vi "Handle Exit.vi"(8 "error in (no error)":errorcluster, 9 "Stop Argument":T1, 10 "Module Admin in":refnum<class "Delacor_lib_QMH_Cloneable Module Admin.lvclass">, 11 "VI reference":refnum<vi>) -> (0 "error out":errorcluster, 3 "Wait for Stop?":bool)   [LabVIEW 2020, in "Counters.lvlib"]
doc: "This VI handles the Exit Message for a DQMH Cloneable module. \n\nThis VI determines if the message was received via the Stop Request or not. If the Exit message was received via the Request Event to Stop the module then there is no need to send the Stop Request again. If it was not, then the Stop Request needs to be fired so the Event Handling Loop can stop.\n\nThis VI also hides the Main.vi Front Panel, this is to ensure that the module stays in memory until the very last step in the Main.vi which is to close the front panel.\n\n_____\nBased on DQMH Project Template 6.1.0.94."
uses:
  Counters.lvlib
  Stop Argument--cluster.ctl
  <vilib>/Delacor/Delacor QMH/Libraries/Cloneable Module Admin_class/Delacor_lib_QMH_Cloneable Module Admin.lvclass
  C:/Program Files (x86)/National Instruments/LabVIEW 2020/vi.lib/Delacor/Delacor QMH/Libraries/Module Admin_class/Delacor_lib_QMH_Module Admin.lvclass
  <vilib>/Delacor/Delacor QMH/Libraries/Cloneable Module Admin_class/Delacor_lib_QMH_Cloneable Module Admin.lvclass/Delacor_lib_QMH_Cloneable Module Admin.ctl
  <vilib>/Delacor/Delacor QMH/Libraries/Module Admin_class/Delacor_lib_QMH_Module Admin.lvclass/Delacor_lib_QMH_Module Admin.ctl
  <vilib>/Delacor/Delacor QMH/Libraries/Cloneable Module Admin_class/Delacor_lib_QMH_Get Module ID.vi
  <vilib>/Delacor/Delacor QMH/Libraries/Module Admin_class/Delacor_lib_QMH_Get External Launch.vi
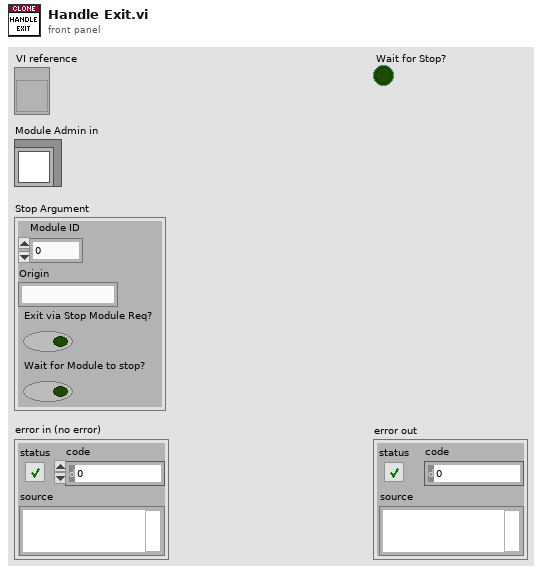
[diagram p1: front panel]
types:
  T1 = typedef "Counters.lvlib/Stop Argument--cluster.ctl" = cluster{"Module ID":i32, "Origin":string, "Exit via Stop Module Req?":bool, "Wait for Module to stop?":bool}
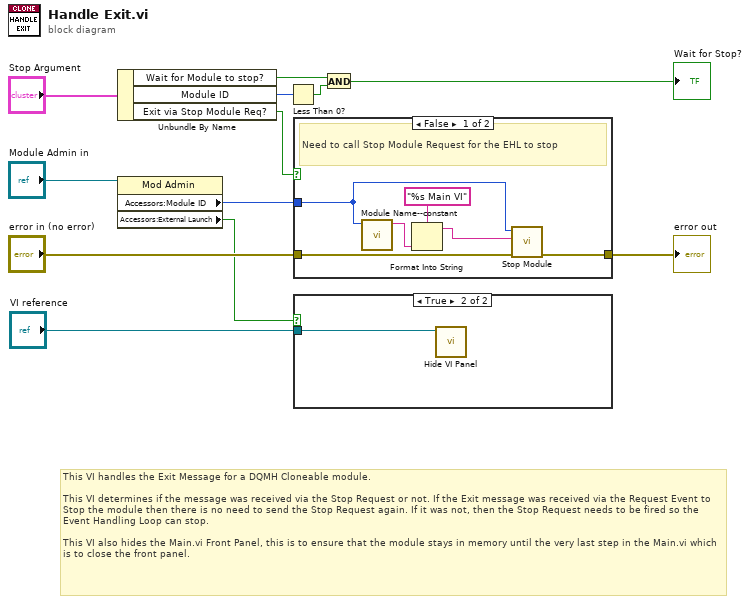
[diagram p0: block diagram]
diagram:
  # "This VI handles the Exit Message for a DQMH Cloneable module. \n\nThis VI determines if the message was received via the Stop Request or not. If the Exit message was received via the Request Event to Stop the module then there is no need to send the Stop Request again. If it was not, then the Stop Request needs to be fired so the Event Handling Loop can stop.\n\nThis VI also hides the Main.vi Front Panel, this is to ensure that the module stays in memory until the very last step in the Main.vi which is to close the front panel."
  n1 = Unbundle By Name("Stop Argument") -> ("Wait for Module to stop?"=w10:bool, "Module ID"=w8:i32, "Exit via Stop Module Req?"=w7:bool)
  n2 = property class="Mod Admin"(reference="Module Admin in") -> ("Accessors:Module ID"=w5:i32, "Accessors:External Launch"=w3:bool)  [unwired: 1 in, 2 out]
  n3 = Less Than 0?(x=w8) -> (x < 0?=w9:bool)
  n4 = case "Exit came from Stop Module Request?" shown="False" w7 {
    tunnel: [w16 w19] -> w1
    tunnel: w5 -> [w14 _]
    tunnel: "error in (no error)" -> [w13 w19]
    frame False {
      # "Need to call Stop Module Request for the EHL to stop"
      n5 = call "Module Name--constant.vi"("Module ID"=w14) -> ("Module Name"=w15:string)  [unwired: 10 in]
      n6 = Format Into String(format string="%s Main VI", w15) -> (resulting string=w17:string)  [unwired: 2 in, 1 out]
      n7 = call "Stop Module.vi"("error in"=w13, "Origin"=w17, "Module ID"=w14) -> ("error out"=w16:errorcluster)  [unwired: 8 in]
    }
    frame True {
      # "no need to call Stop Module Request again."
    }
  }
  "error out" <- w1
  n8 = case shown="True" w3 {
    tunnel: "VI reference" -> [_ w20]
    frame False {
    }
    frame True {
      n9 = call "Hide VI Panel.vi"("VI"=w20) -> ()  [unwired: 10 in, 1 out]
    }
  }
  n10 = And(x=w10, y=w9) -> (x .and. y?=→"Wait for Stop?":bool)
